vi "PicoScope3000aExampleRapidBlock.vi"() -> ()   [LabVIEW 2016]
uses:
  PicoScope3000aLib/PicoScope3000aAnalogChannelSettings.ctl
panel:
  in  "Trigger Settings":T1={"Trigger Enabled"=FALSE, "Trigger Source"=enum."Channel A", "Trigger Threshold (volts)"=0.0, "Trigger Direction"=2, "Trigger Delay (samples)"=0, "Auto Trigger Time (ms)"=1000} {"Trigger Direction" items=["Above", "Below", "Rising", "Falling", "Rising or Falling"]}
  in  "Number of Segments":u32=10
  in  "Rapid Block Acquisition Settings":T2={"preTriggerSamples"=0, "postTriggerSamples"=1000, "timebase"=2, "Down-Sample Mode"=0, "Down Sample Ratio"=1, "Four Channel Device"=FALSE} {"Down Sample Ratio" min=1 step=1; "Down-Sample Mode" items=["None"=0, "Aggregate"=1, "Decimate"=2, "Average"=4]}
  out "Channel A":T3(graph)
  out "Device Info":T4
  out "Properties Panel":T5 {"Max Total Capture Time Available (sec)" format="%.3p"; "Sample Frequency" format="%.3p"; "Sample Rate" format="%.3p"; "Max Samples Available" format="%.3p"; "Total Capture Time (sec)" format="%.3p"}
  in  "Use Serial number":bool
  in  "Batch/Serial":string
  in  "Channel A Settings":T6={"Enabled"=TRUE, "Coupling"=1, "Range"=6, "Analogue Offset"=0.0, "Bandwidth Limit"=0} {"Bandwidth Limit" items=["Full", "20MHz"]; "Range" items=["10 mV", "20 mV", "50 mV", "100 mV", "200 mV", "500 mV", "1 V", "2 V", "5 V", "10 V", "20 V", "50 V ", "100 V"]; "Coupling" items=["AC", "DC"]}
  in  "PS3207A/B device\non non-USB 3.0 Port":bool
  in  "PS34XXA/B\nUSB Powered":bool
  out "Capture Complete":bool
  in  "Run":bool
  in  "Capture Index":u32
  in  "stop":bool
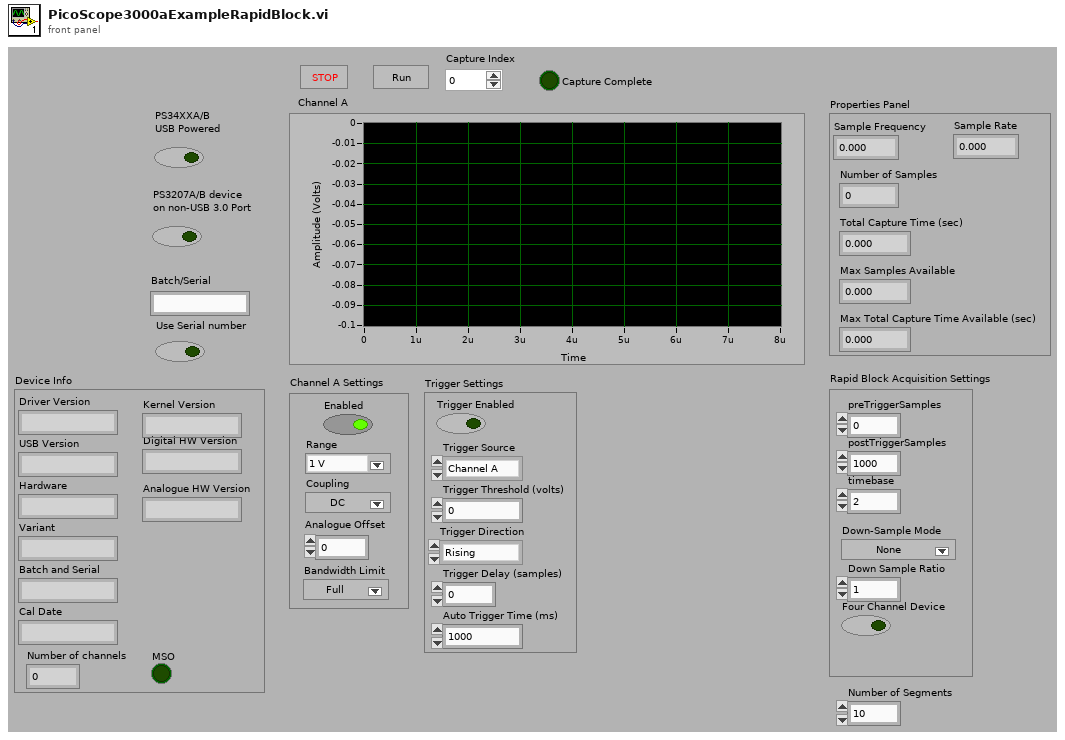
[diagram p1: front panel]
types:
  T1 = cluster{"Trigger Enabled":bool, "Trigger Source":enum32{"Channel A", "Channel B", "Channel C", "Channel D", "Ext."}, "Trigger Threshold (volts)":dbl, "Trigger Direction":u16, "Trigger Delay (samples)":u32, "Auto Trigger Time (ms)":i16}
  T2 = cluster{"preTriggerSamples":u32, "postTriggerSamples":u32, "timebase":u32, "Down-Sample Mode":i32, "Down Sample Ratio":u32, "Four Channel Device":bool}
  T3 = cluster{i32, "Sample Internal":sgl, "Data (Volts)":dbl[]}
  T4 = cluster{"Driver Version":string, "USB Version":string, "Hardware":string, "Variant":string, "Batch and Serial":string, "Cal Date":string, "Kernel Version":string, "Digital HW Version":string, "Analogue HW Version":string, "MSO":bool, "Number of channels":i16}
  T5 = cluster{"Sample Frequency":sgl, "Sample Rate":sgl, "Max Samples Available":i32, "Number of Samples":u32, "Total Capture Time (sec) ":sgl, "Max Total Capture Time Available (sec)":sgl}
  T6 = typedef "PicoScope3000aAnalogChannelSettings.ctl" = cluster{"Enabled":bool, "Coupling":u32, "Range":u32, "Analogue Offset":sgl, "Bandwidth Limit":u32}
  T7 = cluster{"preTriggerSamples":u32, "postTriggerSamples":u32, "timebase":u32, "Down-Sample Mode":i32, "Down Sample Ratio":u32}
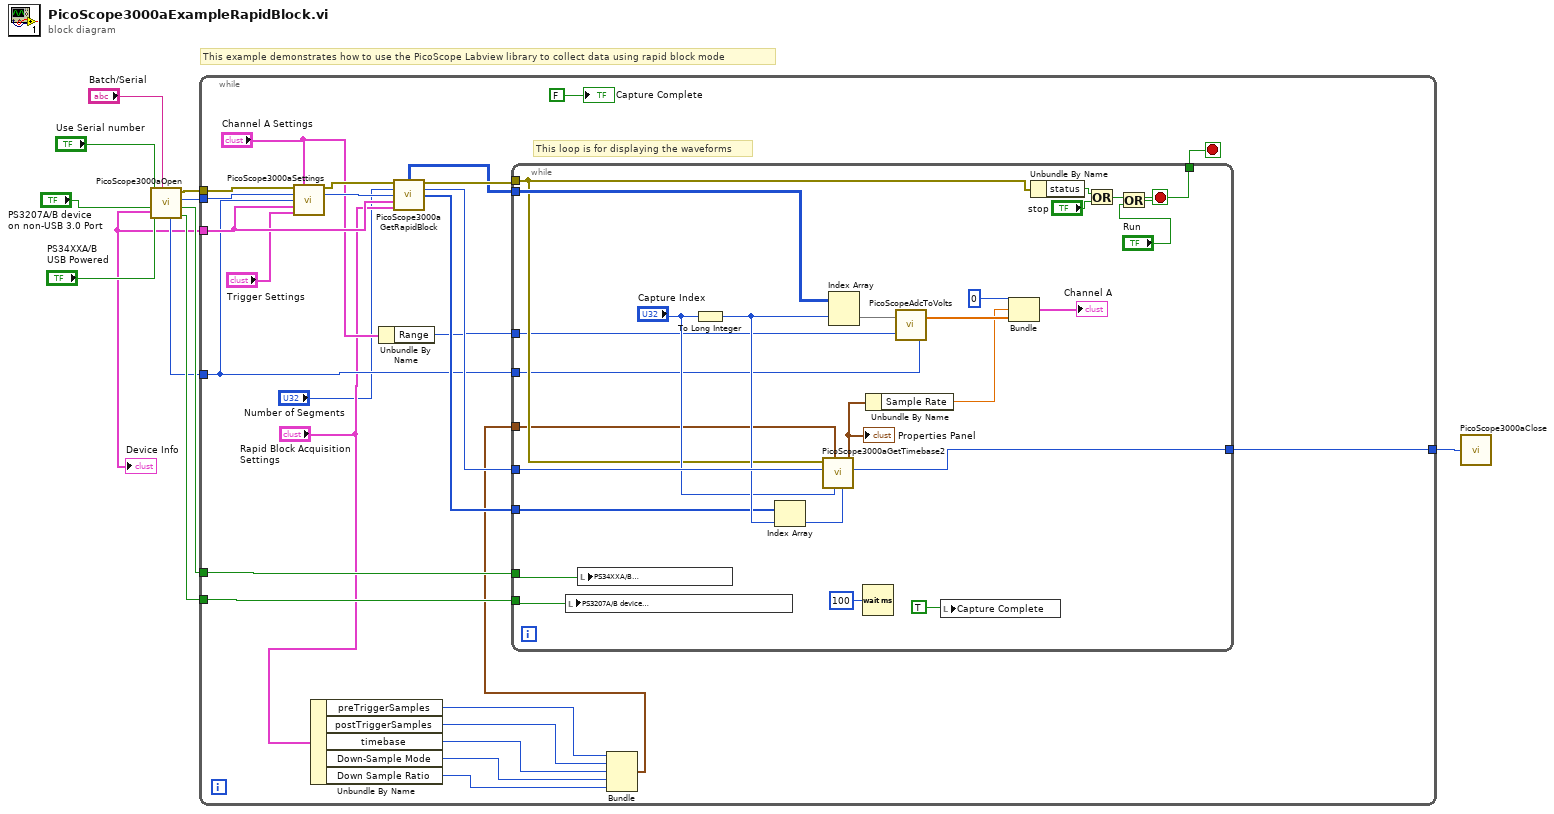
[diagram p0: block diagram]
diagram:
  # "This example demonstrates how to use the PicoScope Labview library to collect data using rapid block mode"
  n1 = call "PicoScope3000aOpen.vi"("Batch/Serial"="Batch/Serial", "USB Powered Control"="PS34XXA/B\nUSB Powered", "USB 3.0 device on non-USB 3.0 Port Control"="PS3207A/B device\non non-USB 3.0 Port", "Use Serial number"="Use Serial number") -> ("USB 3.0 device on non-USB 3.0 Port"=w5:bool, "USB Powered"=w7:bool, "handle"=w9:i16, "error out"=w10:errorcluster, "Max ADC value"=w2:i16, "Device Info"=w1:T4)  [unwired: 2 in]
  "Device Info" <- w1
  n2 = while {
    tunnel: [w28] -> w11
    tunnel: w10 -> [w33]
    tunnel: w9 -> [w32]
    tunnel: w7 -> [w31]
    tunnel: w5 -> [w30]
    tunnel: w1 -> [w25]
    tunnel: w2 -> [w21]
    stop <- w37 stop-if-true
    # "This loop is for displaying the waveforms"
    n3 = call "PicoScope3000aSettings.vi"("error in"=w33, "Channel A Settings"="Channel A Settings", "handle in"=w32, "Max_adc"=w21, "Device Info"=w25, "Trigger Settings"="Trigger Settings") -> ("error out"=w27:errorcluster, "handle out"=w26:i16)  [unwired: 7 in, 1 out]
    n4 = Unbundle By Name("Rapid Block Acquisition Settings") -> ("preTriggerSamples"=w17:u32, "postTriggerSamples"=w20:u32, "timebase"=w19:u32, "Down-Sample Mode"=w16:i32, "Down Sample Ratio"=w14:u32)
    n5 = Unbundle By Name("Channel A Settings") -> ("Range"=w22:u32)
    n6 = call "PicoScope3000aGetRapidBlock.vi"("error in"=w27, "Number of Segments"="Number of Segments", "handle in"=w26, "Device Info"=w25, "Rapid Block Acquisition Settings"="Rapid Block Acquisition Settings") -> ("Channel A Buffer"=w34:i16[][], "error out"=w35:errorcluster, "handle out"=w29:i16, "noOfSamples Array"=w24:u32[])  [unwired: 1 in, 6 out]
    n7 = Bundle("preTriggerSamples"=w17, "postTriggerSamples"=w20, "timebase"=w19, "Down-Sample Mode"=w16, "Down Sample Ratio"=w14) -> (w18:T7)  [unwired: 1 in]
    n8 = while {
      tunnel: [w62] -> w37
      tunnel: w34 -> [w47]
      tunnel: w35 -> [w41]
      tunnel: w31 -> [w56]
      tunnel: w30 -> [w55]
      tunnel: w29 -> [w54]
      tunnel: [w53] -> w28
      tunnel: w24 -> [w45]
      tunnel: w22 -> [w40]
      tunnel: w21 -> [w39]
      tunnel: w18 -> [w38]
      stop <- w61 stop-if-true
      n9 = local write "PS3207A/B device\non non-USB 3.0 Port"(w55) -> ()
      n10 = local write "PS34XXA/B\nUSB Powered"(w56) -> ()
      n11 = To Long Integer(number="Capture Index") -> (32bit integer=w46:i32)
      n12 = Index Array(array=w45, index=w46) -> (element=w52:u32)
      n13 = call "PicoScope3000aGetTimebase2.vi"("Number of Samples"=w52, "Memory Segment"="Capture Index", "Acquisition Settings"=w38, "handle in"=w54, "error in (no error)"=w41) -> ("handle out"=w53:i16, "Properties Panel"=w43:T5)  [unwired: 4 in, 1 out]
      "Properties Panel" <- w43
      n14 = Index Array(array=w47, index (row)=w46) -> (element=w51:i16[])  [unwired: 1 in]
      n15 = Wait (ms)(milliseconds to wait=u32 100) -> ()  [unwired: 1 out]
      n16 = Unbundle By Name(w43) -> ("Sample Rate"=w42:sgl)
      n17 = call "PicoScopeAdcToVolts.vi"("Max_adc"=w39, "Range Index"=w40, "Data"=w51) -> ("Data"=w49:dbl[])
      n18 = local write "Capture Complete"(TRUE ("Capture Complete")) -> ()
      n19 = Bundle(0, "Sample Rate"=w42, "Data"=w49) -> (→"Channel A":cluster{i32, "Sample Rate":sgl, "Data":dbl[]})  [unwired: 1 in]
      n20 = Unbundle By Name(w41) -> ("status"=w57:bool)
      n21 = Or(x=w57, y="stop") -> (x .or. y?=w62:bool)
      n22 = Or(x=w62, y="Run") -> (x .or. y?=w61:bool)
    }
    "Capture Complete" <- FALSE ("Capture Complete")
  }
  n23 = call "PicoScope3000aClose.vi"("handle"=w11) -> ()
